vi "initialise.vi"(8 "error in (no error)":errorcluster, 11 "DL090215DataCollection in":refnum<class "DataCollectionDL091104Scaffold.lvclass">) -> (0 "error out":errorcluster, 3 "DL090215DataCollection out":refnum<class "DataCollectionDL091104Scaffold.lvclass">)   [LabVIEW 2010, in "DataCollectionDL091104Scaffold.lvclass"]
uses:
  DataCollectionDL091104Scaffold.lvclass
  GenericDataCollection/GenericDataCollection/GenericDataCollection.lvclass
  DataCollectionDL091104Scaffold.lvclass/DataCollectionDL091104Scaffold.ctl
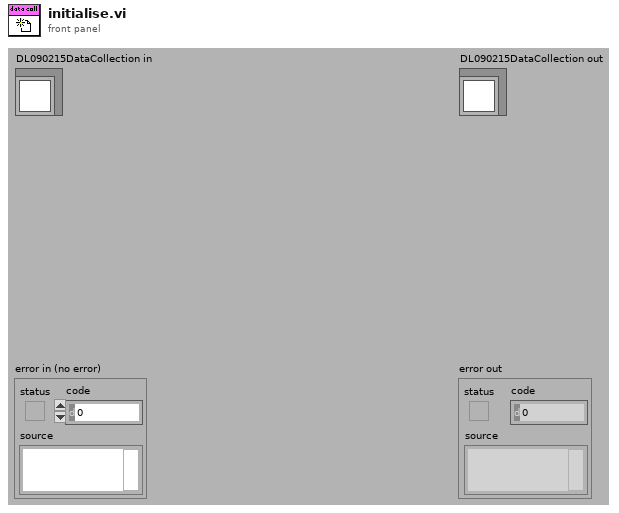
[diagram p1: front panel]
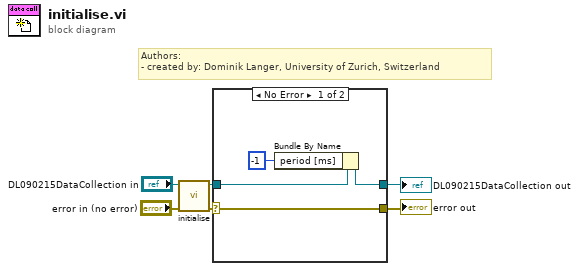
[diagram p0: block diagram]
diagram:
  # "Authors: \n- created by: Dominik Langer, University of Zurich, Switzerland"
  n1 = call-parent "initialise.vi"("error in (no error)"="error in (no error)", "GenericPlugin in"="DL090215DataCollection in") -> ("error out"=w4:errorcluster, "GenericPlugin out"=w3:refnum<class "DataCollectionDL091104Scaffold.lvclass">)  [unwired: 8 out]
  n2 = case shown="No Error" w4 {
    selector: w4 -> [w7 w11]
    tunnel: w3 -> [w8 w12]
    tunnel: [w7 w11] -> w2
    tunnel: [w10 w12] -> w1
    frame No Error {
      n3 = Bundle By Name(cluster=w8, "period [ms]"=-1) -> (w10:refnum<class "DataCollectionDL091104Scaffold.lvclass">)
    }
    frame Error {
    }
  }
  "error out" <- w2
  "DL090215DataCollection out" <- w1
